vi "Apple Gyro Main.vi"(1 "Reset Current":bool, 2 "Reset All":bool, 3 "Override NT?":bool, 4 "Gyro Select (Overide)":enum16{"IMU", "SPI", "Analog", "Navx", "Pigeon"}(ring)=enum."Pigeon") -> (0 "Gyro Yaw Out":dbl format="%#_13g")   [LabVIEW 2016, in "Apple Pi Gyro Library.lvlib"]
uses:
  Apple Pi Gyro Library.lvlib
  <vilib>/Rock Robotics/Network Tables/NT Read Number.vi
  <vilib>/Rock Robotics/Network Tables/NT Write Number.vi
  SimpleGyro ADXRS453/SimpleGyro.lvlib
  ADI MXP IMU/ADI MXP IMU/FRC_ADIS16448_IMU.lvlib
  NavX/navX Library v2/navX Library v2.lvlib
panel:
  out "Pigeon":dbl
  out "Pigeon Active":bool
  out "NavX Active":bool
  out "Analog Active":bool
  out "SPI Active":bool
  out "IMU Active":bool
  out "NavX":dbl
  out "Analog":dbl
  out "IMU":dbl
  out "SPI":dbl
  # "Pull \"Gyro Angle\" from NT for gyro Reading"
  # "Apple Pi 2067 Gyro Library\nBy Chris Garuti\nV 1.0\n\nAllows the selection of 5 different gyrometers through Network Tables"
  # "Active only with Overide on"
  # "All Readings:"
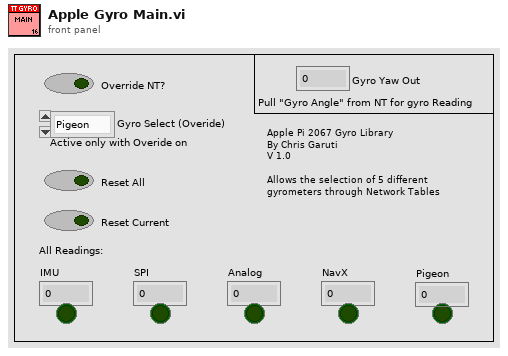
[diagram p1: front panel]
types:
  T1 = typedef "Apple Pi Gyro Library.lvlib/navX Library v2.lvlib/Z900_navX_DeviceTypeDef.ctl" = cluster{"Interface":cluster{"Protocol":T2, "Update Rate (4Hz-100Hz)":u8, "navX Open TypeDef":variant}, "Notify Packet":refnum<notifier>, "Loop VI Refnum":refnum<vi>, "Ready to Close Occurrence Refnum":refnum<k4>}
  T2 = typedef "Apple Pi Gyro Library.lvlib/navX Library v2.lvlib/Z900_navX_ProtocolTypeDef.ctl" = enum16{"SERIAL", "I2C", "SPI"}
  T3 = typedef "Apple Pi Gyro Library.lvlib/FRC_ADIS16448_IMU.lvlib/WPI_IMU_ADIS16448_InterruptDevRef.ctl" = cluster{"ADI IMU DevRef":T4, "InterruptRef":T6}
  T4 = typedef "Apple Pi Gyro Library.lvlib/FRC_ADIS16448_IMU.lvlib/WPI_IMU_ADIS16448_IMUDevRef.ctl" = cluster{"DevStatus":errorcluster, "Handle":i32, "SPI Bus":T5, "Device Found":bool, "Device Ready":bool, "Yaw Axis":enum16{"X", "Y", "Z"}, "AHRS Algorithm":enum16{"Complementary", "Madgwick"}, "Serial":u16, "Lot ID 2":u16, "Lot ID 1":u16, "Product ID":u16}
  T5 = typedef "spi_bus.ctl" = enum16{"SPI On-Board, CS0", "SPI On-Board, CS1", "SPI On-Board, CS2", "SPI On-Board, CS3", "SPI MXP", "Invalid"}
  T6 = typedef "WPI_InterruptRef.ctl" = cluster{"DevStatus":errorcluster, "InterruptIndex":T7}
  T7 = typedef "FPGA_InterruptIndex.ctl" = enum8{"0", "1", "2", "3", "4", "5", "6", "7", "Invalid"}
  T8 = typedef "Apple Pi Gyro Library.lvlib/SimpleGyro.lvlib/WPI_SimpleGyroDevRef.ctl" = cluster{"DevStatus":errorcluster, "Handle":i32, "SPI Bus":T5, "Device Found":bool, "Sample Rate":dbl}
  T9 = typedef "WPI_GyroDevRef.ctl" = cluster{"DevStatus":errorcluster, "Analog Channel":T10, "Offset":dbl, "Gain (VoltsPerDegree/Second)":dbl, "Gyro Type":enum16{"Analog", "XRS450"}, "Handle":i32, "SPI Bus":T5, "Device Found":bool, "Sample Rate":dbl, "Calibrate On Open":bool}
  T10 = typedef "FPGA_AIChannel.ctl" = enum8{"AI 0", "AI 1", "AI 2", "AI 3", "AI MXP 0", "AI MXP 1", "AI MXP 2", "AI MXP 3", "Invalid"}
  T11 = typedef "CTRE_PigeonIMU_DeviceRef.ctl" = cluster{"DeviceStatus":errorcluster, "Device Number":u8, "Type":T12, "Device ID":u32}
  T12 = typedef "CTRE_PigeonIMU_ConnectionType.ctl" = u32
  T13 = cluster{"Yaw":dbl, "Roll":dbl, "Pitch":dbl, "Heading":dbl, "Fused Heading":dbl}
  T14 = typedef "CTRE_PigeonIMU_GlobalStatus.ctl" = cluster{"PigeonState":T15, "FusedHeading":cluster{"Heading":dbl, "Valid?":bool, "Fusing?":bool}, "YPR":cluster{"Yaw":dbl, "Pitch":dbl, "Roll":dbl}, "Compass":cluster{"Heading":dbl, "Magnitude":dbl, "Absolute Heading":dbl}, "Accelerometer":cluster{"Biased":cluster{"X":i16, "Y":i16, "Z":i16, "Norm":i16}, "Angles":cluster{"XZ Tilt":dbl, "YZ Tilt":dbl, "XY Tilt":dbl}}, "Magnetometer":cluster{"Raw":cluster{"X":i16, "Y":i16, "Z":i16}, "Biased":cluster{"X":i16, "Y":i16, "Z":i16}}, "Gyro":cluster{"X":dbl, "Y":dbl, "Z":dbl, "Norm":dbl}, "6D Quaternian":cluster{"W":dbl, "X":dbl, "Y":dbl, "Z":dbl}, "Temp. (C)":dbl, "UpTime":u32, "StartupStatus":cluster{"ResetCount":i32, "ResetFlags":i32, "FirmwareVersion":i32, "HasReset?":bool}, "Calibration":cluster{"CurrentMode":T16, "LastCalError":i32, "CalBooting?":bool}, "CAN Error":errorcluster, "AccumGyro":cluster{"X":dbl, "Y":dbl, "Z":dbl}, "Usage Frame":u32}
  T15 = typedef "CTRE_PigeonIMU_PigeonState.ctl" = enum16{"NoComm", "Initializing", "Ready", "UserCalibration"}
  T16 = typedef "CTRE_PigeonIMU_CalibrationMode.ctl" = u16
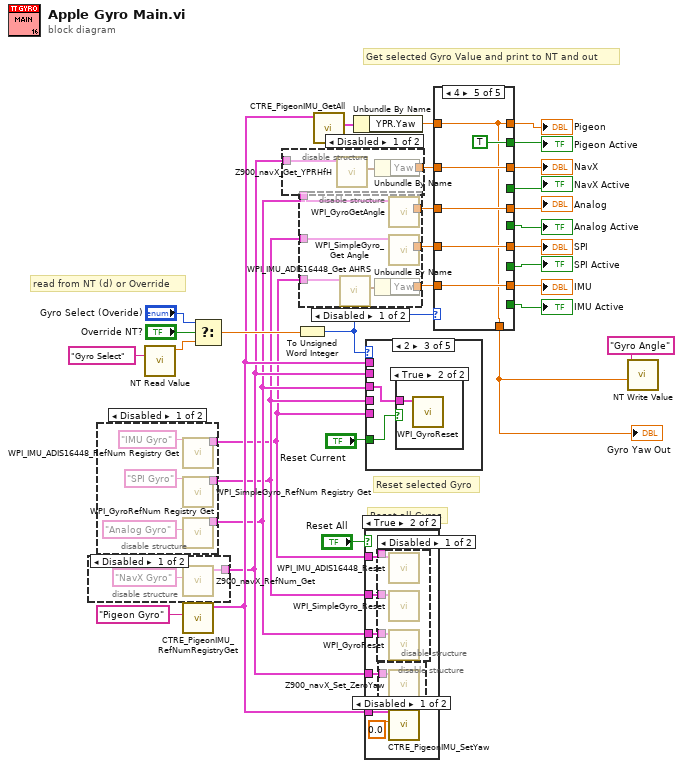
[diagram p0: block diagram]
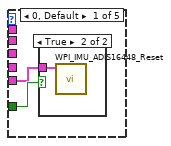
[diagram p9: hidden frame]
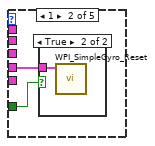
[diagram p11: hidden frame]
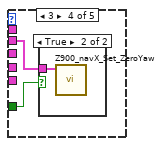
[diagram p14: hidden frame]
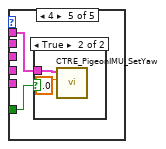
[diagram p16: hidden frame]
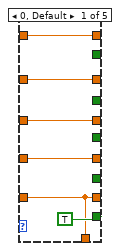
[diagram p18: hidden frame]
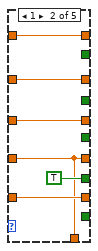
[diagram p19: hidden frame]
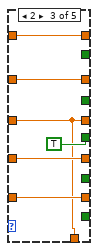
[diagram p20: hidden frame]
diagram:
  # "Get selected Gyro Value and print to NT and out"
  # "read from NT (d) or Override"
  # "Reset all Gyros"
  # "Reset selected Gyro"
  n1 = disable-structure shown="Disabled" {
    disable-tunnel: [w33 _] -> w6
    frame Disabled {
      n2 = call "Z900_navX_RefNum_Get.vi"("refnum name"="NavX Gyro") -> ("navX Device"=w33:T1)  [unwired: 9 in, 1 out]
    }
    frame Enabled {
    }
  }
  n3 = disable-structure shown="Disabled" {
    disable-tunnel: [w37 _] -> w5
    disable-tunnel: [w36 _] -> w4
    disable-tunnel: [w35 _] -> w3
    frame Disabled {
      n4 = call "WPI_IMU_ADIS16448_RefNum Registry Get.vi"("refnum name"="IMU Gyro") -> ("ADI IMU Interrupt DevRef"=w35:T3)  [unwired: 9 in, 1 out]
      n5 = call "WPI_SimpleGyro_RefNum Registry Get.vi"("refnum name"="SPI Gyro") -> ("SimpleGyroDevRef"=w36:T8)  [unwired: 9 in, 1 out]
      n6 = call <vilib>:"WPI_GyroRefNum Registry Get.vi"("refnum name"="Analog Gyro") -> ("GyroDevRef"=w37:T9)  [unwired: 9 in, 1 out]
    }
    frame Enabled {
    }
  }
  n7 = call-poly <vilib>:"NT Read Value.vi"("Name"="Gyro Select") -> ("Numeric"=w30:dbl)  [unwired: 9 in, 1 out]
  n8 = call <vilib>:"CTRE_PigeonIMU_RefNumRegistryGet.vi"("refnum name"="Pigeon Gyro") -> ("PigeonIMUDevRef"=w7:T11)  [unwired: 9 in, 1 out]
  n9 = Select(t="Gyro Select (Overide)", s="Override NT?", f=w30) -> (s? t:f=w20:dbl)
  n10 = disable-structure shown="Disabled" {
    disable-tunnel: [w42 _] -> w17
    disable-tunnel: w6 -> [w41 _]
    frame Disabled {
      n11 = call "Z900_navX_Get_YPRHfH.vi"("navX Device"=w41) -> ("YRPHfH"=w43:T13)  [unwired: 7 in, 3 out]
      n12 = Unbundle By Name(w43) -> ("Yaw"=w42:dbl)
    }
    frame Enabled {
    }
  }
  n13 = To Unsigned Word Integer(number=w20) -> (unsigned 16bit integer=w28:u16)
  n14 = disable-structure shown="Disabled" {
    disable-tunnel: [w49 _] -> w16
    disable-tunnel: [w48 _] -> w15
    disable-tunnel: [w47 _] -> w14
    disable-tunnel: w5 -> [w46 _]
    disable-tunnel: w4 -> [w45 _]
    disable-tunnel: w3 -> [w44 _]
    frame Disabled {
      n15 = call "WPI_IMU_ADIS16448_Get AHRS.vi"("ADI IMU Interrupt DevRef"=w44) -> ("IMU AHRS Out"=w50:cluster{"Pitch":dbl, "Roll":dbl, "Yaw":dbl})  [unwired: 6 in, 4 out]
      n16 = Unbundle By Name(w50) -> ("Yaw"=w47:dbl)
      n17 = call <vilib>:"WPI_GyroGetAngle.vi"("GyroDevRef"=w46) -> ("Angle"=w49:dbl)  [unwired: 6 in, 4 out]
      n18 = call "WPI_SimpleGyro_Get Angle.vi"("SimpleGyroDevRef"=w45) -> ("Angle"=w48:dbl)  [unwired: 7 in, 3 out]
    }
    frame Enabled {
    }
  }
  n19 = call <vilib>:"CTRE_PigeonIMU_GetAll.vi"("PigeonIMUDevRef"=w7) -> ("Get All"=w2:T14)  [unwired: 8 in, 2 out]
  n20 = Unbundle By Name(w2) -> ("YPR.Yaw"=w18:dbl)
  n21 = case shown="True" "Reset All" {
    tunnel: w3 -> [_ w56]
    tunnel: w4 -> [_ w55]
    tunnel: w5 -> [_ w54]
    tunnel: w6 -> [_ w53]
    tunnel: w7 -> [_ w52]
    frame False {
    }
    frame True {
      n22 = disable-structure shown="Disabled" {
        disable-tunnel: w56 -> [w60 _]
        disable-tunnel: w55 -> [w59 _]
        disable-tunnel: w54 -> [w58 _]
        frame Disabled {
          n23 = call "WPI_IMU_ADIS16448_Reset.vi"("ADI IMU Interrupt DevRef"=w60) -> ()  [unwired: 9 in, 2 out]
          n24 = call "WPI_SimpleGyro_Reset.vi"("SimpleGyroDevRef"=w59) -> ()  [unwired: 9 in, 2 out]
          n25 = call <vilib>:"WPI_GyroReset.vi"("GyroDevRef"=w58) -> ()  [unwired: 9 in, 2 out]
        }
        frame Enabled {
        }
      }
      n26 = disable-structure shown="Disabled" {
        disable-tunnel: w53 -> [w57 _]
        frame Disabled {
          n27 = call "Z900_navX_Set_ZeroYaw.vi"("navX Device"=w57) -> ()  [unwired: 9 in, 2 out]
        }
        frame Enabled {
        }
      }
      n28 = call <vilib>:"CTRE_PigeonIMU_SetYaw.vi"("Value"=0.0, "PigeonIMUDevRef"=w52) -> ()  [unwired: 8 in, 2 out]
    }
  }
  n29 = case shown="2" w28 {
    tunnel: "Reset Current" -> [w62 w65 w67 w70 w74]
    tunnel: w3 -> [w61 _ _ _ _]
    tunnel: w4 -> [_ w64 _ _ _]
    tunnel: w5 -> [_ _ w68 _ _]
    tunnel: w6 -> [_ _ _ w71 _]
    tunnel: w7 -> [_ _ _ _ w73]
    frame 0, Default {
      n30 = case shown="True" w62 {
        tunnel: w61 -> [_ w63]
        frame False {
        }
        frame True {
          n31 = call "WPI_IMU_ADIS16448_Reset.vi"("ADI IMU Interrupt DevRef"=w63) -> ()  [unwired: 9 in, 2 out]
        }
      }
    }
    frame 1 {
      n32 = case shown="True" w65 {
        tunnel: w64 -> [_ w66]
        frame False {
        }
        frame True {
          n33 = call "WPI_SimpleGyro_Reset.vi"("SimpleGyroDevRef"=w66) -> ()  [unwired: 9 in, 2 out]
        }
      }
    }
    frame 2 {
      n34 = case shown="True" w67 {
        tunnel: w68 -> [_ w69]
        frame False {
        }
        frame True {
          n35 = call <vilib>:"WPI_GyroReset.vi"("GyroDevRef"=w69) -> ()  [unwired: 9 in, 2 out]
        }
      }
    }
    frame 3 {
      n36 = case shown="True" w70 {
        tunnel: w71 -> [_ w72]
        frame False {
        }
        frame True {
          n37 = call "Z900_navX_Set_ZeroYaw.vi"("navX Device"=w72) -> ()  [unwired: 9 in, 2 out]
        }
      }
    }
    frame 4 {
      n38 = case shown="True" w74 {
        tunnel: w73 -> [_ w76]
        frame False {
        }
        frame True {
          n39 = call <vilib>:"CTRE_PigeonIMU_SetYaw.vi"("Value"=0.0, "PigeonIMUDevRef"=w76) -> ()  [unwired: 8 in, 2 out]
        }
      }
    }
  }
  n40 = case shown="4" w28 {
    tunnel: [_ _ _ TRUE _] -> w24
    tunnel: [_ _ TRUE _ _] -> w23
    tunnel: [_ TRUE _ _ _] -> w22
    tunnel: [TRUE _ _ _ _] -> w21
    tunnel: [w80 w83 w89 w95 w101] -> w19
    tunnel: w18 -> [w81 w87 w93 w99 w101]
    tunnel: w17 -> [w77 w86 w90 w95 w103]
    tunnel: w16 -> [w78 w85 w89 w96 w104]
    tunnel: w15 -> [w79 w83 w91 w97 w105]
    tunnel: w14 -> [w80 w84 w92 w98 w106]
    tunnel: [w81 w87 w93 w99 w101] -> w13
    tunnel: [w77 w86 w90 w95 w103] -> w12
    tunnel: [w78 w85 w89 w96 w104] -> w11
    tunnel: [w79 w83 w91 w97 w105] -> w10
    tunnel: [w80 w84 w92 w98 w106] -> w9
    tunnel: [_ _ _ _ TRUE] -> w8
    frame 0, Default {
    }
    frame 1 {
    }
    frame 2 {
    }
    frame 3 {
    }
    frame 4 {
    }
  }
  "Gyro Yaw Out" <- w19
  "NavX" <- w12
  "NavX Active" <- w24
  "IMU Active" <- w21
  "SPI" <- w10
  "IMU" <- w9
  "Analog Active" <- w23
  "SPI Active" <- w22
  "Analog" <- w11
  "Pigeon" <- w13
  "Pigeon Active" <- w8
  n41 = call-poly <vilib>:"NT Write Value.vi"("Numeric"=w19, "Name"="Gyro Angle") -> ()  [unwired: 9 in, 1 out]
